vi "GetUnitInformation.vi"(0 "handle in":i32, 1 "UnitAddress(0)":u16, 2 "ResponseAddress(0)":u8, 5 "error in":errorcluster) -> (14 "handle out":i32, 15 "FirmwareRevision":u8, 16 "ResetFlag":u8, 17 "Temperature":i16, 18 "SerialNumber":u16, 19 "error out":errorcluster)   [LabVIEW 2014, in "Sixpack - Driver.lvlib"]
doc: "Dieser Befehl ermöglicht die Abfrage der Firmware-Revision, Reset-Flag, Temperatur und Seriennummer.\n\nCMD $43\nResponseAdress: Adresse des Host zum empfangen der Antwort\n\nAntwort\n\nFirmwareRevision : (z.B. 164=V1.6.4)\nRESETFLAG: Ist beim ersten Auslesen 1, hinterher 0\nTemperature: Temperatur auf dem PACK in °C\nSerialNumber: Seriennummer des PACK"
uses:
  Sixpack - Driver.lvlib
  DLL/PackDLL.dll
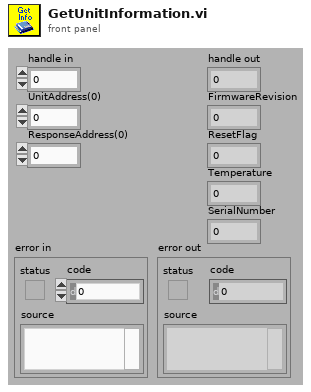
[diagram p1: front panel]
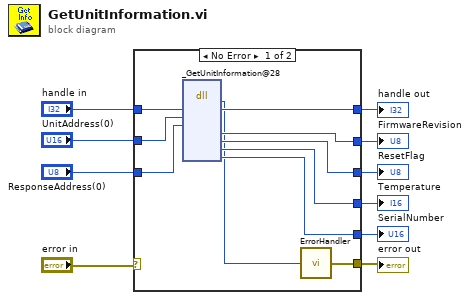
[diagram p0: block diagram]
diagram:
  n1 = case shown="No Error" "error in" {
    selector: "error in" -> [_ w21]
    tunnel: "handle in" -> [w20 w22]
    tunnel: [w19 w22] -> w9
    tunnel: "UnitAddress(0)" -> [w18 _]
    tunnel: "ResponseAddress(0)" -> [w17 _]
    tunnel: [w16 _] -> w6
    tunnel: [w15 _] -> w5
    tunnel: [w14 _] -> w4
    tunnel: [w13 _] -> w3
    tunnel: [w11 w21] -> w2
    frame No Error {
      n2 = dll-call lib="D:/CS-Source/LV2014/GPL/instr.lib/SixPack/PackDLL/DLL/PackDLL.dll" fn="_GetUnitInformation@28" label="GetUnitInformation"("HANDLE"=w20, "UnitAddress"=w18, "ResponseAddress"=w17) -> ("BOOLEAN"=w12:i8, "HANDLE"=w19:i32, "FirmwareRevision"=w13:u8, "ResetFlag"=w16:u8, "Temperature"=w15:i16, "SerialNumber"=w14:u16)  [unwired: 9 in, 2 out]
      n3 = call "ErrorHandler.vi"("BOOLEAN"=w12) -> ("error out"=w11:errorcluster)
    }
    frame Error {
    }
  }
  "handle out" <- w9
  "FirmwareRevision" <- w3
  "ResetFlag" <- w6
  "Temperature" <- w5
  "SerialNumber" <- w4
  "error out" <- w2
